vi "receive.vi"(8 "error in":errorcluster {"code" format="Error %.0f"}, 10 "nats message":T1, 11 "NATS Subscriber in":refnum<class "NATS Subscription.lvclass">) -> (0 "error out":errorcluster {"code" format="Error %.0f"}, 3 "NATS Subscriber out":refnum<class "NATS Subscription.lvclass">)   [LabVIEW 2024, in "NATS Subscription.lvlib" / "NATS Subscription.lvclass"]
uses:
  NATS Subscription.lvclass
  Controls/nats message.ctl
  Controls/msg type.ctl
  NATS Subscription.lvclass/NATS Subscription.ctl
  get reply queue.vi
  NATS Core.lvlib
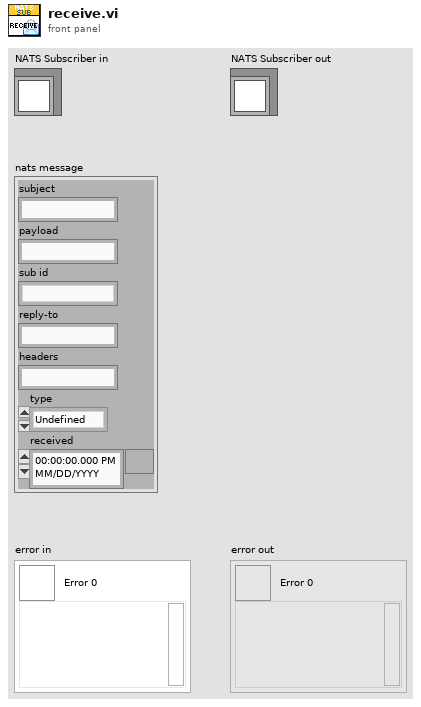
[diagram p1: front panel]
types:
  T1 = typedef "NATS Core.lvlib/nats message.ctl" = cluster{"subject":string, "payload":string, "sub id":string, "reply-to":string, "headers":string, "type":T2, "received":timestamp}
  T2 = typedef "NATS Core.lvlib/msg type.ctl" = enum16{"Undefined", "MSG", "HMSG", "+OK", "PING", "PONG", "-ERR", "INFO"}
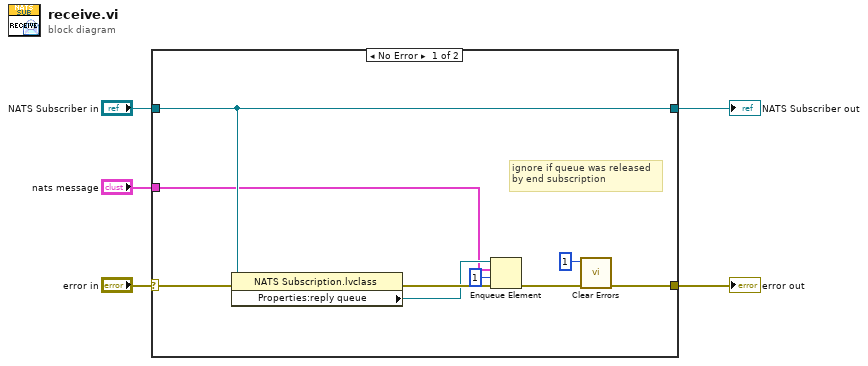
[diagram p0: block diagram]
diagram:
  n1 = case shown="No Error" "error in" {
    selector: "error in" -> [w12 w16]
    tunnel: [w8 w16] -> w4
    tunnel: [w11 w15] -> w2
    tunnel: "NATS Subscriber in" -> [w11 w15]
    tunnel: "nats message" -> [w10 _]
    frame No Error {
      # "ignore if queue was released\nby end subscription"
      n2 = property on="Property Node" class="NATS Subscription.lvclass"(reference=w11, error in=w12) -> (error out=w14:errorcluster, "Properties:reply queue"=w13:refnum<queue>)  [unwired: 1 out]
      n3 = Enqueue Element(queue=w13, element=w10, timeout in ms (-1)=1, error in (no error)=w14) -> (error out=w9:errorcluster)  [unwired: 2 out]
      n4 = call <vilib>:"Clear Errors.vi"("error in (no error)"=w9, "specific error code to clear (0: all)"=1) -> ("error out"=w8:errorcluster)  [unwired: 4 in, 1 out]
    }
    frame Error {
    }
  }
  "error out" <- w4
  "NATS Subscriber out" <- w2
